vi "AMI.vi"(0 "VISA resource name":refnum<visa-resource-name>, 11 "error in":errorcluster) -> (4 "VISA resource name out":refnum<visa-resource-name>, 6 "Information":string, 8 "Model Name":string, 10 "Version-Revision":string, 15 "error out":errorcluster)   [LabVIEW 2017, in "Samwontech TEMP2xxx.lvlib"]
doc: "AMI Command is used to get the controller own information"
uses:
  <instrlib>/Samwontech TEMP2xxx/Samwontech TEMP2xxx.lvlib
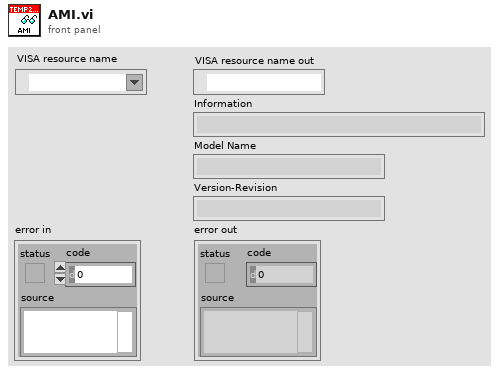
[diagram p1: front panel]
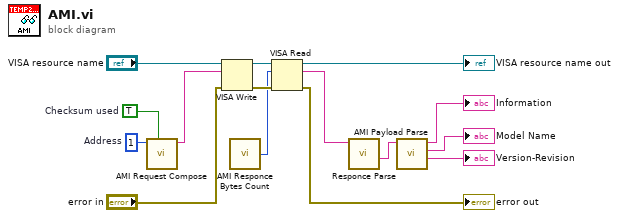
[diagram p0: block diagram]
diagram:
  w14 = TRUE  # Checksum used
  w15 = u8 1  # Address
  n1 = call <instrlib>:"AMI Request Compose.vi"("Checksum used"=w14, "Address"=w15) -> ("Request"=w10:string)  [unwired: 9 in]
  n2 = VISA Write(VISA resource name="VISA resource name", write buffer=w10, error in (no error)="error in") -> (VISA resource name out=w12:refnum<visa-resource-name>, error out=w13:errorcluster)  [unwired: 1 out]
  n3 = call <instrlib>:"AMI Responce Bytes Count.vi"() -> ("Bytes Count"=w7:u32)
  n4 = VISA Read(VISA resource name=w12, byte count=w7, error in (no error)=w13) -> (VISA resource name out=→"VISA resource name out":refnum<visa-resource-name>, read buffer=w6:string, error out=→"error out":errorcluster)  [unwired: 1 out]
  n5 = call <instrlib>:"Responce Parse.vi"("Responce"=w6) -> ("Payload"=w5:string)  [unwired: 8 in, 2 out]
  n6 = call <instrlib>:"AMI Payload Parse.vi"("Payload"=w5) -> ("Version-Revision"=→"Version-Revision":string, "Model Name"=→"Model Name":string, "Information"=→"Information":string)  [unwired: 8 in]
